vi "CLC_CTTC_L3_InPhaseCal.vi"() -> ()   [LabVIEW 2023, in "Clover_Cell.lvlib"]
uses:
  Clover_Cell.lvlib
  lib/Anritsu Signal Analyzer Series/Anritsu Signal Analyzer Series.lvlib
  <vilib>/Utility/file.llb/Write Delimited Spreadsheet (DBL).vi
panel:
  in  "WaitingTime":u32=500
  in  "AiP_Change":u16(ring)=1 items=["AiP_1"=1, "AiP_2"=2, "AiP_3"=3, "AiP_4"=4]
  in  "AiP_Base":u16(ring)=1 items=["AiP_1"=1, "AiP_2"=2, "AiP_3"=3, "AiP_4"=4]
  in  "Polarity":u16(ring) items=["H", "V"]
  in  "AvgTimes":i32=5
  in  "TRXmode":u16(ring)=1 items=["Rx"=2, "Tx"=1]
  in  "FileName_Note":string
  out "AiP_Base_Ch":i32
  out "AiP_Change_OFFSetPhase":i32
  out "AiP_Change_Ch":i32
  out "max index\n(OFFSet Step)":i32
  out "trmode":u16
  in  "VISA resource name":refnum<visa-resource-name>="TCPIP0::172.16.1.100::inst0::INSTR"
  out "FileNAME_Dual":string
  out "OK?":bool
  out "output cluster":T1={"address"="192.168.100.111", "remote port or service name"=5025, "timeout ms (60000)"=10000}
  out "SA1":dbl[](graph)
  out "error out":errorcluster
  # "CTTC Gen3 L3 256 in-Phase Calibration with SA"
  # "Setting"
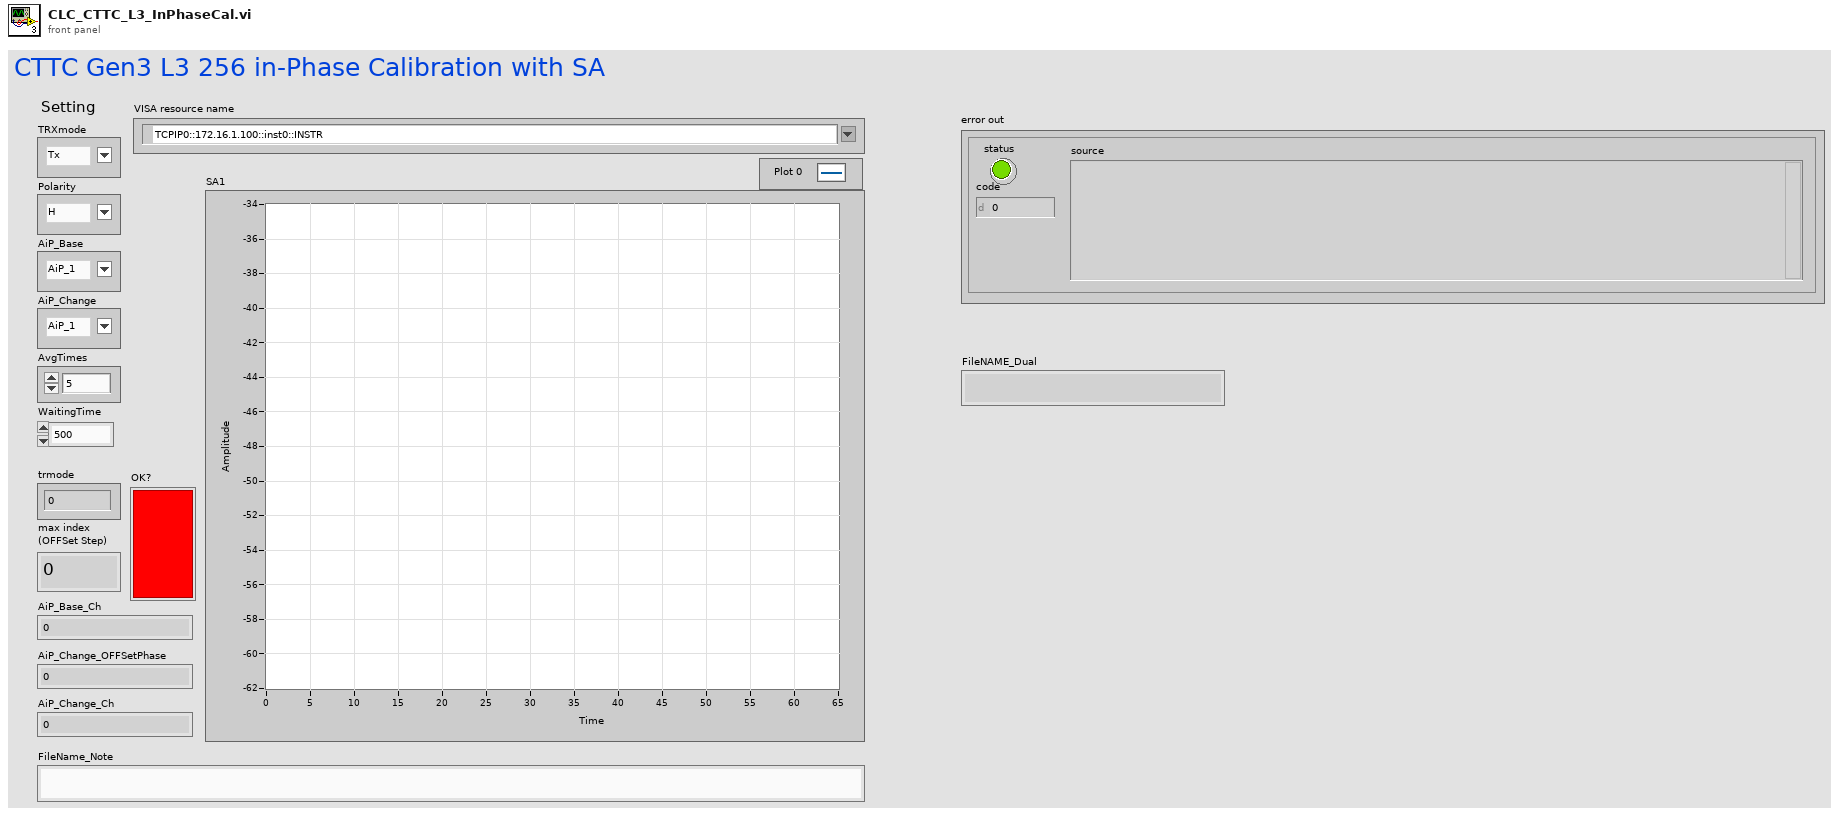
[diagram p1: front panel]
types:
  T1 = cluster{"address":string, "remote port or service name":u16, "timeout ms (60000)":i32}
  T2 = cluster{"Mode":u16, "Polarity":u16, "CH_ON/OFF":u16, "Channel":i32, "Gain":i32, "Phase":i32}
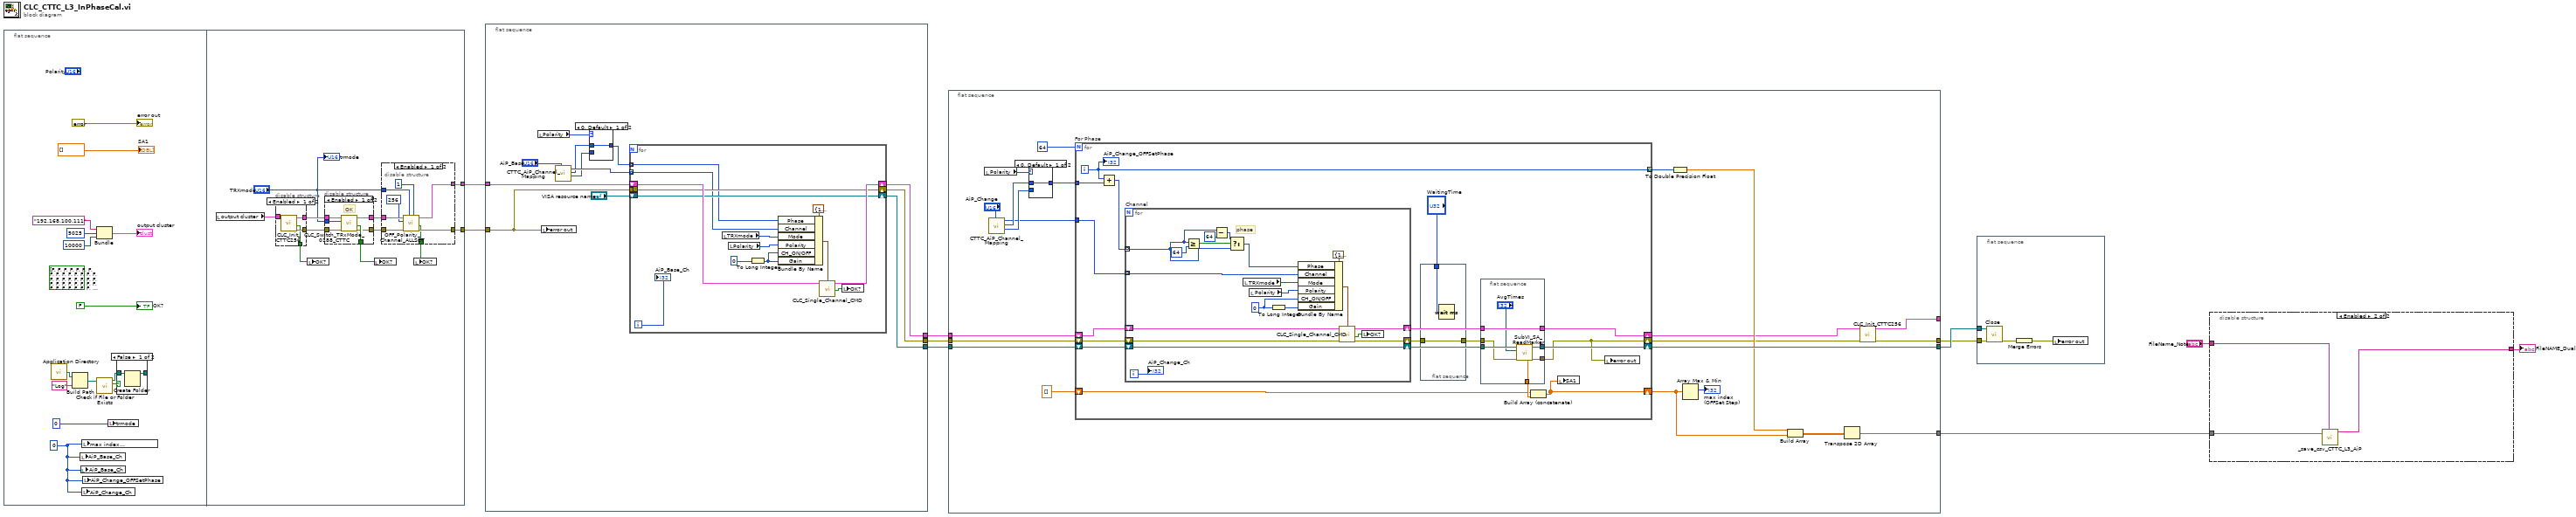
[diagram p0: block diagram]
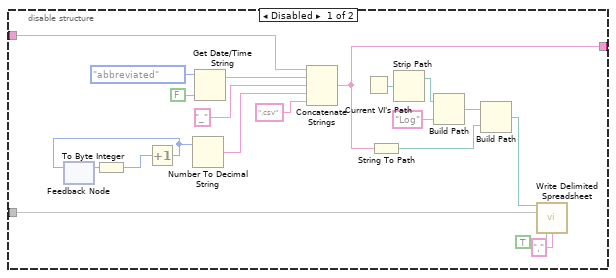
[diagram p4: hidden frame]
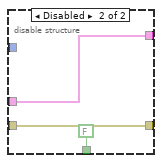
[diagram p6: hidden frame]
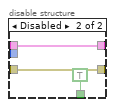
[diagram p7: hidden frame]
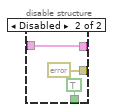
[diagram p8: hidden frame]
diagram:
  n1 = flat-sequence {
    tunnel: [w28] -> w1
    tunnel: [w33] -> w2
    frame #0 {
      w11 = 0 ("max index\n(OFFSet Step)")
      (unwired) bool[][] [[FALSE, FALSE, FALSE, FALSE, FALSE, FALSE, FALSE, FALSE], [FALSE, FALSE, FALSE, FALSE, FALSE, FALSE, FALSE, FALSE], [FALSE, FALSE, FALSE, FALSE, FALSE, FALSE, FALSE, FALSE], [FALSE, FALSE, FALSE, FALSE, FALSE, FALSE, FALSE, FALSE], [FALSE, FALSE, FALSE, FALSE, FALSE, FALSE, FALSE, FALSE], [FALSE, FALSE, FALSE, FALSE, FALSE, FALSE, FALSE, FALSE], [FALSE, FALSE, FALSE, FALSE, FALSE, FALSE, FALSE, FALSE], [FALSE, FALSE, FALSE, FALSE, FALSE, FALSE, FALSE, FALSE]] ("Operating \nChannel(s)")
      n2 = call <vilib>:"Application Directory.vi"() -> ("Application Directory"=w16:path)
      n3 = Build Path(base path=w16, name or relative path="Log") -> (appended path=w13:path)
      n4 = local write "AiP_Base_Ch"(w11) -> ()
      n5 = local write "AiP_Base_Ch"(w11) -> ()
      n6 = local write "AiP_Change_Ch"(w11) -> ()
      n7 = local write "max index\n(OFFSet Step)"(w11) -> ()
      n8 = local write "AiP_Change_OFFSetPhase"(w11) -> ()
      n9 = Bundle("address"="192.168.100.111", "remote port or service name"=u16 5025, "timeout ms (60000)"=10000) -> (→"output cluster":T1)  [unwired: 1 in]
      n10 = call <vilib>:"Check if File or Folder Exists.vi"("path"=w13) -> ("file or folder exists?"=w15:bool, "dup path"=w14:path)  [unwired: 8 in, 1 out]
      n11 = local write "trmode"(u16 0 ("trmode")) -> ()
      n12 = case shown="False" w15 {
        tunnel: w14 -> [w26 w27]
        tunnel: [w25 w27] -> _
        frame False {
          n13 = Create Folder(path (use dialog)=w26) -> (created path=w25:path)  [unwired: 2 in, 2 out]
        }
        frame True {
        }
      }
      "error out" <- errorcluster {"status"=FALSE, "code"=0, "source"=""} ("error out")
      "OK?" <- FALSE ("OK?")
      "SA1" <- dbl[] []
    }
    frame #1 {
      n14 = local read "output cluster"() -> (w38:T1)
      n15 = disable-structure shown="Enabled" {
        disable-tunnel: w38 -> [w62 w65]
        disable-tunnel: [w61 w65] -> w37
        disable-tunnel: [w60 errorcluster {"status"=FALSE, "code"=0, "source"=""} ("error in (no error)")] -> w35
        disable-tunnel: [w59 TRUE ("OK?")] -> w30
        frame Enabled {
          n16 = call "CLC_Init_CTTC256.vi"("TCPIPin"=w62) -> ("error out"=w60:errorcluster, "Status"=w59:bool, "TCPIPin 2"=w61:T1)  [unwired: 8 in]
        }
        frame Disabled {
        }
      }
      n17 = local write "OK?"(w30) -> ()
      n18 = disable-structure shown="Enabled" {
        disable-tunnel: w37 -> [w55 w57]
        disable-tunnel: [w54 TRUE ("OK?")] -> w36
        disable-tunnel: w35 -> [w53 w56]
        disable-tunnel: [w52 w56] -> w34
        disable-tunnel: [w51 w57] -> w32
        disable-tunnel: "TRXmode" -> [w50 _]
        frame Enabled {
          # "OK"
          n19 = call "CLC_Switch_TRxMode_0188_CTTC.vi"("error in (no error)"=w53, "Text Ring"=w50, "TCPIPin"=w55) -> ("error out"=w52:errorcluster, "OK?"=w54:bool, "TCPIPin 2"=w51:T1)  [unwired: 6 in]
        }
        frame Disabled {
        }
      }
      n20 = local write "OK?"(w36) -> ()
      n21 = disable-structure shown="Enabled" {
        disable-tunnel: w34 -> [w46 w48]
        disable-tunnel: [w45 w48] -> w33
        disable-tunnel: w32 -> [w44 w47]
        disable-tunnel: [w43 FALSE ("OK?")] -> w31
        disable-tunnel: "TRXmode" -> [w41 _]
        disable-tunnel: [w39 w47] -> w28
        frame Enabled {
          n22 = call "OFF_Polarity_Channel_ALLSET.vi"("CH_ON:0/OFF:1"=u16 1, "Mode"=w41, "error in"=w46, "Channel"=256, "TCPIPin"=w44) -> ("error out"=w45:errorcluster, "OK?"=w43:bool, "TCPIPout"=w39:T1)  [unwired: 4 in]
        }
        frame Disabled {
        }
      }
      n23 = local write "OK?"(w31) -> ()
      "trmode" <- "TRXmode"
    }
  }
  n24 = flat-sequence {
    tunnel: [w77] -> w10
    tunnel: [w76] -> w9
    tunnel: [w75] -> w8
    tunnel: w2 -> [w74]
    tunnel: w1 -> [w72]
    frame #0 {
      n25 = local read "Polarity"() -> (w70:u16)
      n26 = local write "error out"(w74) -> ()
      n27 = call "CTTC_AiP_Channel_Mapping.vi"("AiP"="AiP_Base") -> ("Pol_V"=w67:i32[], "Pol_H"=w68:i32[], "Ch_Index"=w69:i32[])  [unwired: 8 in]
      n28 = case shown="0, Default" w70 {
        tunnel: w68 -> [w78 _]
        tunnel: [w78 w79] -> w66
        tunnel: w67 -> [_ w79]
        frame 0, Default {
        }
        frame 1 {
        }
      }
      n29 = for {
        shift-right: [w90] -> w75
        shift-left: w72 -> [w89]
        tunnel: w74 -> [w84]
        shift-right: [w84] -> w76
        shift-left: _ -> [_]
        shift-right: [w83] -> w77
        shift-left: "VISA resource name" -> [w83]
        tunnel: w69 -> [w82] mode=indexing
        tunnel: w66 -> [w81] mode=indexing
        i -> [w80]
        n30 = local read "TRXmode"() -> (w87:u16)
        n31 = local read "Polarity"() -> (w86:u16)
        n32 = To Long Integer(number=u16 0 ("CH_ON/OFF")) -> (32bit integer=w85:i32)
        n33 = Bundle By Name(cluster=T2 {"Mode"=1, "Polarity"=1, "CH_ON/OFF"=1, "Channel"=0, "Gain"=0, "Phase"=0} ("Channel params"), "Phase"=w81, "Channel"=w82, "Mode"=w87, "Polarity"=w86, "CH_ON/OFF"=w85, "Gain"=w85) -> (w93:T2)
        n34 = call "CLC_Single_Channel_CMD.vi"("Channel params"=w93, "TCPIPin"=w89) -> ("OK?"=w92:bool, "TCPIPout"=w90:T1)  [unwired: 7 in, 1 out]
        n35 = local write "OK?"(w92) -> ()
        "AiP_Base_Ch" <- w80
      }
    }
  }
  n36 = flat-sequence {
    tunnel: w10 -> [w115]
    tunnel: w9 -> [w114]
    tunnel: w8 -> [w113]
    tunnel: [w98] -> w5
    tunnel: [w111] -> w4
    tunnel: [w94] -> w3
    tunnel: [w96] -> _
    frame #0 {
      n37 = local read "Polarity"() -> (w107:u16)
      n38 = call "CTTC_AiP_Channel_Mapping.vi"("AiP"="AiP_Change") -> ("Pol_V"=w105:i32[], "Pol_H"=w106:i32[], "Ch_Index"=w104:i32[])  [unwired: 8 in]
      n39 = case shown="0, Default" w107 {
        tunnel: w106 -> [w116 _]
        tunnel: [w116 w117] -> w103
        tunnel: w105 -> [_ w117]
        frame 0, Default {
        }
        frame 1 {
        }
      }
      n40 = for "For Phase" {
        N: 64 -> [_]
        shift-right: [w129] -> w97
        shift-left: w113 -> [w131]
        shift-right: [w128] -> w95
        shift-left: w114 -> [w132]
        shift-right: [w135] -> w111
        shift-left: w115 -> [w126]
        shift-right: [w130] -> w102
        shift-left: dbl[] [] -> [w133]
        tunnel: w104 -> [w124]
        tunnel: w103 -> [w123]
        tunnel: [w121] -> w100 mode=indexing
        i -> [w121]
        n41 = Add(x=w121, y=w123) -> (x+y=w122:i32[])
        n42 = for "Channel" {
          shift-right: [w147] -> w120
          shift-left: w132 -> [w152]
          shift-right: [w148] -> w127
          shift-left: w131 -> [w151]
          shift-right: [w146] -> w125
          shift-left: w126 -> [w146]
          tunnel: w124 -> [w145] mode=indexing
          tunnel: w122 -> [w140] mode=indexing
          i -> [w138]
          w156 = u16 0 ("CH_ON/OFF")
          # "phase"
          n43 = Greater Or Equal?(x=w140, y=64) -> (x >= y?=w143:bool)
          n44 = Subtract(x=w140, y=64) -> (x-y=w144:i32)
          n45 = Select(t=w144, s=w143, f=w140) -> (s? t:f=w139:i32)
          n46 = local read "TRXmode"() -> (w154:u16)
          n47 = local read "Polarity"() -> (w155:u16)
          n48 = To Long Integer(number=w156) -> (32bit integer=w157:i32)
          n49 = Bundle By Name(cluster=T2 {"Mode"=1, "Polarity"=1, "CH_ON/OFF"=1, "Channel"=0, "Gain"=0, "Phase"=0} ("Channel params"), "Phase"=w139, "Channel"=w145, "Mode"=w154, "Polarity"=w155, "CH_ON/OFF"=w156, "Gain"=w157) -> (w149:T2)
          n50 = call "CLC_Single_Channel_CMD.vi"("Channel params"=w149, "error in"=w152, "TCPIPin"=w151) -> ("error out"=w147:errorcluster, "OK?"=w150:bool, "TCPIPout"=w148:T1)  [unwired: 6 in]
          n51 = local write "OK?"(w150) -> ()
          "AiP_Change_Ch" <- w138
        }
        n52 = flat-sequence {
          tunnel: w120 -> [w137]
          tunnel: [w137] -> w119
          tunnel: "WaitingTime" -> [w136]
          frame #0 {
            n53 = Wait (ms)(milliseconds to wait=w136) -> ()  [unwired: 1 out]
          }
        }
        n54 = flat-sequence {
          tunnel: [w164] -> w135
          tunnel: [w163] -> w134
          tunnel: [w162] -> w128
          tunnel: w125 -> [w161]
          tunnel: w119 -> [w160]
          tunnel: [w159] -> w129
          tunnel: w127 -> [w159]
          frame #0 {
            n55 = call "SubVI_SA_ReadMarker.vi"("error in (no error)"=w160, "AvgTimes"="AvgTimes", "VISA resource name"=w161) -> ("error out"=w162:errorcluster, "VISA resource name out"=w164:refnum<visa-resource-name>, "Marker Power"=w163:dbl)  [unwired: 5 in, 1 out]
          }
        }
        n56 = Build Array (concatenate)(w133, w134) -> (w130:dbl[])
        n57 = local write "SA1"(w130) -> ()
        n58 = local write "error out"(w128) -> ()
        "AiP_Change_OFFSetPhase" <- w121
      }
      n59 = To Double Precision Float(number=w100) -> (double precision float=w99:dbl[])
      n60 = Array Max & Min(array=w102) -> (max index (indices)=→"max index\n(OFFSet Step)":i32)  [unwired: 3 out]
      n61 = Build Array(w99, w102) -> (w112:dbl[][])
      n62 = Transpose 2D Array(2D array=w112) -> (transposed array=w98:dbl[][])
      n63 = call "CLC_Init_CTTC256.vi"("error in (no error)"=w95, "TCPIPin"=w97) -> ("error out"=w94:errorcluster, "TCPIPin 2"=w96:T1)  [unwired: 7 in, 1 out]
    }
  }
  n64 = flat-sequence {
    tunnel: w4 -> [w167]
    tunnel: w3 -> [w166]
    frame #0 {
      n65 = call "Close.vi"("error in (no error)"=w166, "VISA resource name"=w167) -> ("error out"=w168:errorcluster)  [unwired: 9 in]
      n66 = Merge Errors(w168) -> (w165:errorcluster)
      n67 = local write "error out"(w165) -> ()
    }
  }
  n68 = disable-structure shown="Enabled" {
    disable-tunnel: [w187 w189] -> w7
    disable-tunnel: "FileName_Note" -> [w183 w190]
    disable-tunnel: w5 -> [w182 w191]
    frame Disabled {
      n69 = feedback #1() -> (w181:i8)  [unwired: 1 in]
      n70 = To Byte Integer(number=w181) -> (8bit integer=w179:i8)
      n71 = Increment(x=w179) -> (x+1=w180:i8)
      n72 = feedback-in #1(w180) -> ()
      n73 = Number To Decimal String(number=w180) -> (decimal integer string=w178:string)  [unwired: 1 in]
      n74 = Get Date/Time String(date format (0)=enum16{"short", "long", "abbreviated"}."abbreviated", want seconds? (F)=FALSE) -> (date string=w188:string)  [unwired: 1 in, 1 out]
      n75 = Concatenate Strings(w183, w188, "_" ("delimiter (\\t)"), w178, ".csv" ("delimiter (\\t)")) -> (w187:string)
      n76 = Current VI's Path() -> (path=w173:path)
      n77 = String To Path(string=w187) -> (path=w172:path)
      n78 = Strip Path(path=w173) -> (stripped path=w174:path)  [unwired: 1 out]
      n79 = Build Path(base path=w174, name or relative path="Log") -> (appended path=w176:path)
      n80 = Build Path(base path=w176, name or relative path=w172) -> (appended path=w171:path)
      n81 = call-poly <vilib>:"Write Delimited Spreadsheet.vi"("file path (dialog if empty)"=w171, "2D data"=w182, "transpose? (no:F)"=TRUE, "delimiter (\\t)"="," ("delimiter (\\t)")) -> ()  [unwired: 10 in, 2 out]
    }
    frame Enabled {
      n82 = call "_save_csv_CTTC_L3_AiP.vi"("delimiter (\\t)"=w190, "Data"=w191) -> ("FileName"=w189:string)  [unwired: 9 in]
    }
  }
  "FileNAME_Dual" <- w7
